vi "ex9-1.vi"() -> ()   [LabVIEW 2013]
uses:
  <vilib>/NXT/Block Support/NXT_InputPort.ctl
  <vilib>/NXT/Dual Mode Library/Sensors/EV3_Ultrasonic_CM.vi
  <vilib>/NXT/Dual Mode Library/Sensors/EV3_Touch_Pressed.vi
  <vilib>/NXT/Dual Mode Library/Sensors/EV3_Gyro_Angle.vi
  <vilib>/NXT/Dual Mode Library/Sensors/EV3_Color_Ambient.vi
  <vilib>/NXT/Dual Mode Library/Sensors/EV3_Color_Reflect.vi
panel:
  out "Waveform Chart":sgl(graph)
  out "Degrees":sgl
  in  "Port (Port 1) 4":T1 items=["Port 1", "Port 2", "Port 3", "Port 4"]
  in  "Boolean":bool
  out "Tank":dbl(slide) scale=0.0..100.0
  out "Scaled Value":sgl
  in  "Port (Port 1) 3":T1 items=["Port 1", "Port 2", "Port 3", "Port 4"]
  out "0, 1":i16
  out "Yes / No":bool
  in  "Port (Port 1) 2":T1 items=["Port 1", "Port 2", "Port 3", "Port 4"]
  out "Gauge":dbl(knob) scale=0.0..255.0
  out "Centimeters":sgl
  in  "Port (Port 1)":T1 items=["Port 1", "Port 2", "Port 3", "Port 4"]
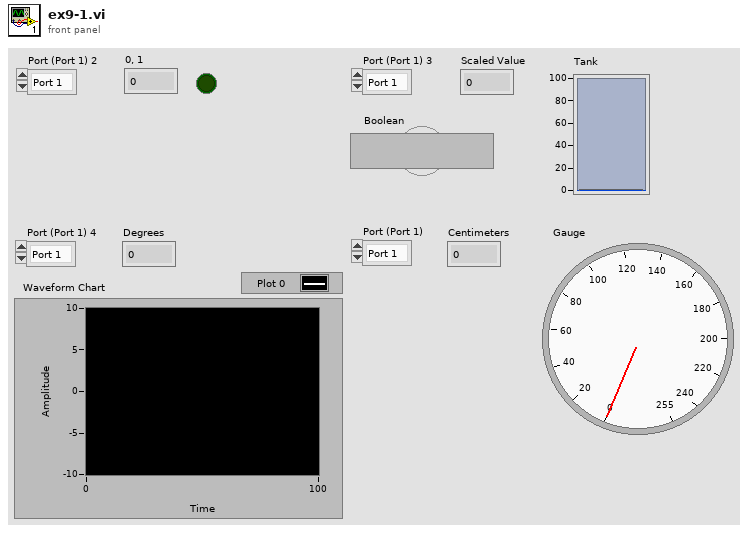
[diagram p1: front panel]
types:
  T1 = typedef "NXT_InputPort.ctl" = u32
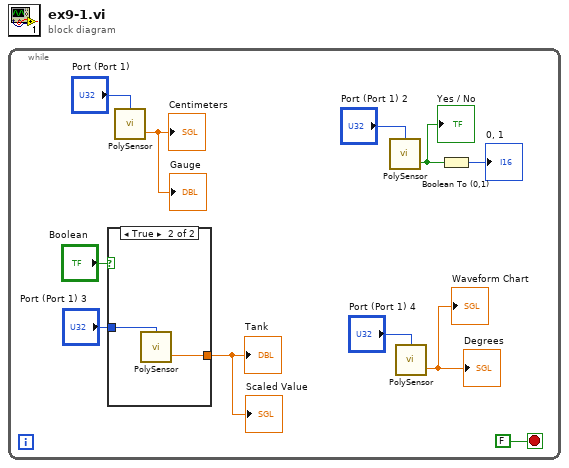
[diagram p0: block diagram]
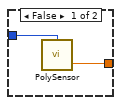
[diagram p2: hidden frame]
diagram:
  n1 = while {
    stop <- FALSE stop-if-true
    n2 = case shown="True" "Boolean" {
      tunnel: "Port (Port 1) 3" -> [w12 w15]
      tunnel: [w13 w14] -> w5
      frame False {
        n3 = call-poly <vilib>:"PolySensor.vi"("Port (Port 1)"=w12) -> ("Scaled Value"=w13:sgl)  [unwired: 2 in, 1 out]
      }
      frame True {
        n4 = call-poly <vilib>:"PolySensor.vi"("Port (Port 1)"=w15) -> ("Scaled Value"=w14:sgl)  [unwired: 2 in, 1 out]
      }
    }
    "Scaled Value" <- w5
    "Tank" <- w5
    n5 = call-poly <vilib>:"PolySensor.vi"("Port (Port 1)"="Port (Port 1)") -> ("Centimeters"=→"Centimeters" →"Gauge":sgl)  [unwired: 2 in, 1 out]
    n6 = call-poly <vilib>:"PolySensor.vi"("Port (Port 1)"="Port (Port 1) 2") -> ("Pressed"=w8:bool)  [unwired: 2 in, 1 out]
    "Yes / No" <- w8
    n7 = call-poly <vilib>:"PolySensor.vi"("Port (Port 1)"="Port (Port 1) 4") -> ("Degrees"=→"Degrees" →"Waveform Chart":sgl)  [unwired: 2 in, 1 out]
    n8 = Boolean To (0,1)(Boolean=w8) -> (0, 1=→"0, 1":i16)
  }
